vi "main_SUBVi.vi"() -> ()   [LabVIEW 2020]
panel:
  in  "Enum":enum16{"add", "sub", "mul", "div"}(ring)
  out "ans":dbl
  in  "B":dbl
  in  "A":dbl
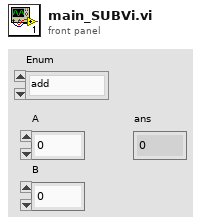
[diagram p1: front panel]
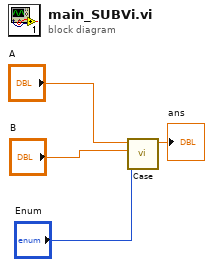
[diagram p0: block diagram]
diagram:
  n1 = call "Case.vi"("Enum"="Enum", "B"="B", "A"="A") -> ("ans"=→"ans":dbl)  [unwired: 8 in]
